vi "UMLEditor saveIniFileInfo.vi"(1 "localVariables":T2 {"ObjectHotspots"."HotSpot"."y" format="%.2f"; "ObjectHotspots"."HotSpot"."x" format="%.2f"; "NodesBounds"."height" format="%.2f"; "NodesBounds"."width" format="%.2f"; "NodesBounds"."y" format="%.2f"; "NodesBounds"."x" format="%.2f"; "offset"."y" format="%.2f"; "offset"."x" format="%.2f"; "gridSize" format="%.2f"; "dragStartBounds"."height" format="%.2f"; "dragStartBounds"."width" format="%.2f"; "dragStartBounds"."y" format="%.2f"; "dragStartBounds"."x" format="%.2f"; "dragStartPoint"."y" format="%.2f"; "dragStartPoint"."x" format="%.2f"; "rubberBandStart"."y" format="%.2f"; "rubberBandStart"."x" format="%.2f"; "lastMousePoint"."y" format="%.2f"; "lastMousePoint"."x" format="%.2f"; "zoom" format="%.2f"}, 5 "error in (no error)":errorcluster, 6 "diagramType":T1) -> (19 "error out":errorcluster)   [LabVIEW 2014]
doc: "Gets current diagram values"
uses:
  <resource>/Framework/Providers/Open_GDS/UML/UMLEditor/UMLEditor LocalVariablesType.ctl
  <resource>/Framework/Providers/Open_GDS/UML/Graphics_class/Graphics.lvclass
  <resource>/Framework/Providers/Open_GDS/UML/Grid_class/Grid.lvclass
  <resource>/Framework/Providers/Open_GDS/UML/AbstractEdge_class/AbstractEdge.lvclass
  <resource>/Framework/Providers/Open_GDS/UML/AbstractNode_class/AbstractNode.lvclass
  <resource>/Framework/Providers/Open_GDS/UML/UMLEditor/UMLEditor statesType.ctl
  <resource>/Framework/Providers/Open_GDS/UML/UMLEditor/UMLEditor tooltype.ctl
  <resource>/Framework/Providers/Open_GDS/UML/UMLEditor/UMLEditor toolsType.ctl
  <resource>/Framework/Providers/Open_GDS/UML/Graph_class/private/diagramType.ctl
  <resource>/Framework/Providers/Open_GDS/UML/Graph_class/Graph.lvclass
  <resource>/Framework/Providers/Open_GDS/UML/General/Point/Point Point2D.ctl
  <resource>/Framework/Providers/Open_GDS/UML/General/Rectangle/Rectangle Rectangle2D.ctl
  <resource>/Framework/Providers/Open_GDS/UML/UMLEditor/UMLEditor ExportType.ctl
  <resource>/Framework/Providers/Open_GDS/UML/UMLEditor/UMLEditor FlattenCommandType.ctl
  <resource>/Framework/Providers/Open_GDS/UML/UMLEditor/UMLEditor ExecuteCommandType.ctl
  <resource>/Framework/Providers/Open_GDS/UML/ContextHelp/ContextHelp_EventType.ctl
  <resource>/Framework/Providers/Open_GDS/UML/UMLEditor/UMLEditor_HotSpotData.ctl
  <resource>/Framework/Providers/Open_GDS/UML/UMLEditor/UMLEditor_HotSpotType.ctl
  <resource>/Framework/Providers/Open_GDS/UML/UmlEditor_class/EventData.ctl
  <resource>/Framework/Providers/Open_GDS/UML/UMLEditor/UMLEditor_IniFileData.ctl
  <resource>/Framework/Providers/Open_GDS/UML/UMLEditor/UMLEditor_SyncOptions.ctl
  <resource>/Framework/Providers/Open_GDS/UML/UMLEditor/UMLEditor_StoredPathes.ctl
  <resource>/Framework/Providers/Open_GDS/UML/UMLEditor/UMLEditor_StoredColors.ctl
  <resource>/Framework/Providers/Open_GDS/UML/UmlEditor_class/UmlEditor.lvclass
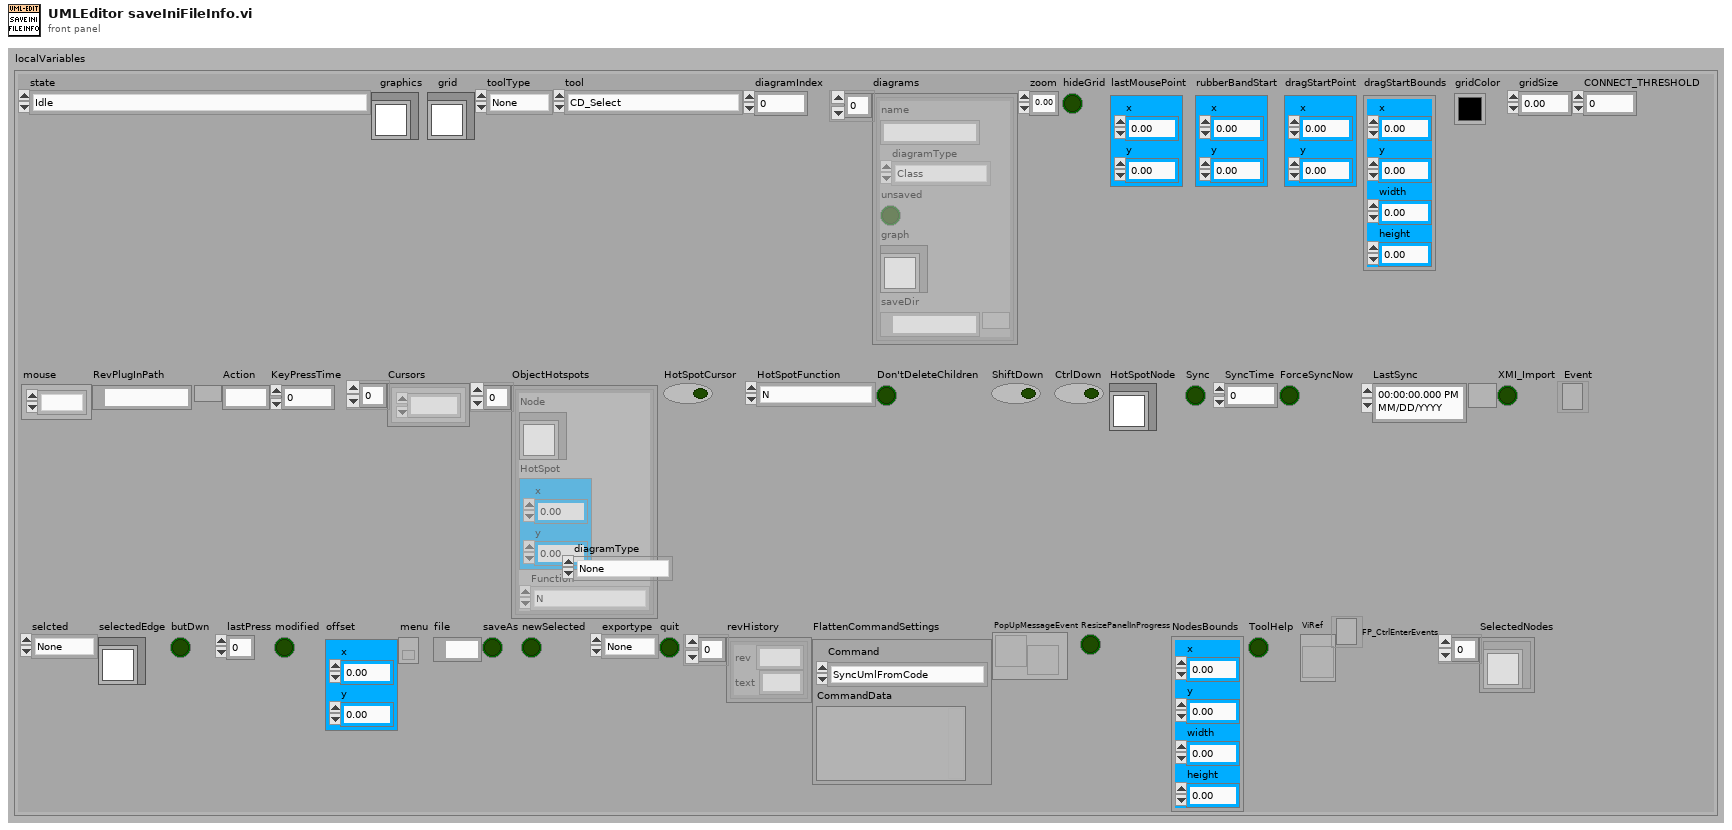
[diagram p1: front panel]
types:
  T1 = typedef "Graph.lvclass/diagramType.ctl" = enum16{"None", "Class", "Sequency", "State", "UseCase", "DQMH-Module"}
  T2 = typedef "UMLEditor LocalVariablesType.ctl" = cluster{"state":T3, "graphics":refnum<class "Graphics.lvclass">, "grid":refnum<class "Grid.lvclass">, "toolType":T4, "tool":T5, "diagramIndex":i32, "diagrams":cluster{"name":string, "diagramType":T1, "unsaved":bool, "graph":refnum<class "Graph.lvclass">, "saveDir":path}[], "zoom":dbl, "hideGrid":bool, "lastMousePoint":T6, "rubberBandStart":T6, "dragStartPoint":T6, "dragStartBounds":T7, "gridColor":u32, "gridSize":dbl, "CONNECT_THRESHOLD":i32, "selcted":T4, "selectedEdge":refnum<class "AbstractEdge.lvclass">, "butDwn":bool, "lastPress":u32, "modified":bool, "offset":T6, "menu":refnum<k9>, "file":path, "saveAs":bool, "newSelected":bool, "exportype":T8, "quit":bool, "revHistory":cluster{"rev":string, "text":string}[], "FlattenCommandSettings":T9, "PopUpMessageEvent":T11, "ResizePanelInProgress":bool, "NodesBounds":T7, "ToolHelp":bool, "ViRef":refnum<vi>, "FP_CtrlEnterEvents":refnum<event-registration>, "SelectedNodes":refnum<class "AbstractNode.lvclass">[], "mouse":refnum<k1>, "RevPlugInPath":path, "Action":string, "KeyPressTime":u32, "Cursors":refnum<k1>[], "ObjectHotspots":T12[], "HotSpotCursor":bool, "HotSpotFunction":T13, "Don'tDeleteChildren":bool, "ShiftDown":bool, "CtrlDown":bool, "HotSpotNode":refnum<class "AbstractNode.lvclass">, "Sync":bool, "SyncTime":u32, "ForceSyncNow":bool, "LastSync":timestamp, "XMI_Import":bool, "Event":refnum<event-registration>}
  T3 = typedef "UMLEditor statesType.ctl" = enum16{"Idle", "CheckLicense", "revHistory", "Init", "Init2", "EditSelected", "RemoveSelected", "PaintComponent", "ChangeZoom", "ChangeGridSize", "Open", "Close", "Save", "ExportPicture", "Export", "Repaint", "Error", "Exit", "QUIT", "CreateScript", "ExecuteScript", "ClassReversedEngineering", "PlugInReverseEngineering", "StateReversedEngineering", "AutoPlace", "ExecuteCommand", "OpenClass", "SyncAll", "StraightenAssociation", "Copy", "Paste", "AddNodeFromProjectTree", "AddNodeFromProjectTree+SyncAll", "PanAndRepaint", "Init3", "CopyPaste", "ApplyDesignPattern", "AnalyseViInStateDiagram", "AutoSync"}
  T4 = typedef "UMLEditor tooltype.ctl" = enum16{"None", "Node", "Edge"}
  T5 = typedef "UMLEditor toolsType.ctl" = enum16{"CD_Select", "CD_Class", "CD_Interface", "CD_Package", "CD_Note", "CD_Dependency", "CD_Inheritance", "CD_InterfaceImp", "CD_Association", "CD_Aggregation", "CD_Composite", "CD_NoteConn", "SQD_Select", "SQD_Object", "SQD_ActionBar", "SQD_Note", "SQD_Call", "SQD_NoteConn", "UD_Select", "UD_System", "UD_Actor", "UD_UseCase", "UD_Note", "UD_Assoiciation", "UD_Generalization", "UD_GeneralizationIncludes", "UD_GeneralizationExtends", "UD_Realization", "UD_Relationship", "UD_NoteEdge", "STD_Select", "STD_State", "STD_InitailState", "STD_FinalState", "STD_ChoiseState", "STD_StateTransation", "STD_Note", "STD_NoteEdge", "DM_Select", "DM_VI", "DM_Module", "DM_Request", "DM_RequestWait", "DM_Roundtrip", "DM_Broadcast", "DM_Note", "DM_NoteEdge"}
  T6 = typedef "Point Point2D.ctl" = cluster{"x":dbl, "y":dbl}
  T7 = typedef "Rectangle Rectangle2D.ctl" = cluster{"x":dbl, "y":dbl, "width":dbl, "height":dbl}
  T8 = typedef "UMLEditor ExportType.ctl" = enum16{"None", "Printer", "png", "jpg", "roseUML"}
  T9 = typedef "UMLEditor FlattenCommandType.ctl" = cluster{"Command":T10, "CommandData":variant}
  T10 = typedef "UMLEditor ExecuteCommandType.ctl" = enum16{"SyncUmlFromCode", "SyncCodeFromUML", "OpenClass", "OpenFile", "CreateClass", "CreateVI", "OpenClassAttribute", "LocateInProject"}
  T11 = typedef "ContextHelp_EventType.ctl" = refnum<user-event>
  T12 = typedef "UMLEditor_HotSpotData.ctl" = cluster{"Node":refnum<class "AbstractNode.lvclass">, "HotSpot":T6, "Function":T13}
  T13 = typedef "UMLEditor_HotSpotType.ctl" = enum16{"N", "NE", "E", "SE", "S", "SW", "W", "NW", "Expand", "Collaps"}
  T14 = typedef "UMLEditor_IniFileData.ctl" = cluster{"RecentFiles":string[], "LastDiagramType":T1, "ShowToolHelp":bool, "Paths":cluster{"LastSerachPath":path, "QueuedArrayStateVI":path, "ClassBasePath":path, "VITemplatePath":path, "ApplicationTemplatePath":path, "RevPlugIns":path}, "Colors":cluster{"ClassBackgroudColor":u32, "ClassBackgroudColorWithClassPath":u32, "ClassBackgroudColorForApplicationVIStereotype":u32, "ClassBackgroudColorForTypeStereotype":u32, "StateBackgroudColor":u32}, "ProjectBaseClassOption":bool, "CreateTypesWhenSynchronizing":bool, "AttributeToIgnoreInSync":string[], "ToolTip":cluster{"ToolTipOpen":bool, "LastToolTip":i32}, "ClassesToIgnoreInSync":string[], "UndoSize":i32, "OpenLastSavedFile":bool, "SyncOption":T15, "SyncTime":u32, "Params":cluster{"Name":string, "Value":string}[]}
  T15 = typedef "UMLEditor_SyncOptions.ctl" = cluster{"IgnoreInstrLib":bool, "IgnoreUserLib":bool, "IgnoreViLib":bool}
  T16 = typedef "UMLEditor_StoredPathes.ctl" = enum16{"LastSearchPath", "QueuedArrayStateVI", "ClassBasePath", "ViTemplatePath", "ApplicationTemplatePath", "IniFilePath", "WizDir", "RevPlugInPath"}
  T17 = typedef "UMLEditor_StoredColors.ctl" = enum16{"ClassBackgroudColor", "ClassBackgroudColorWithClassPath", "ClassBackgroudColorForApplicationVIStereotype", "ClassBackgroudColorForTypeStereotype", "StateBackgroudColor"}
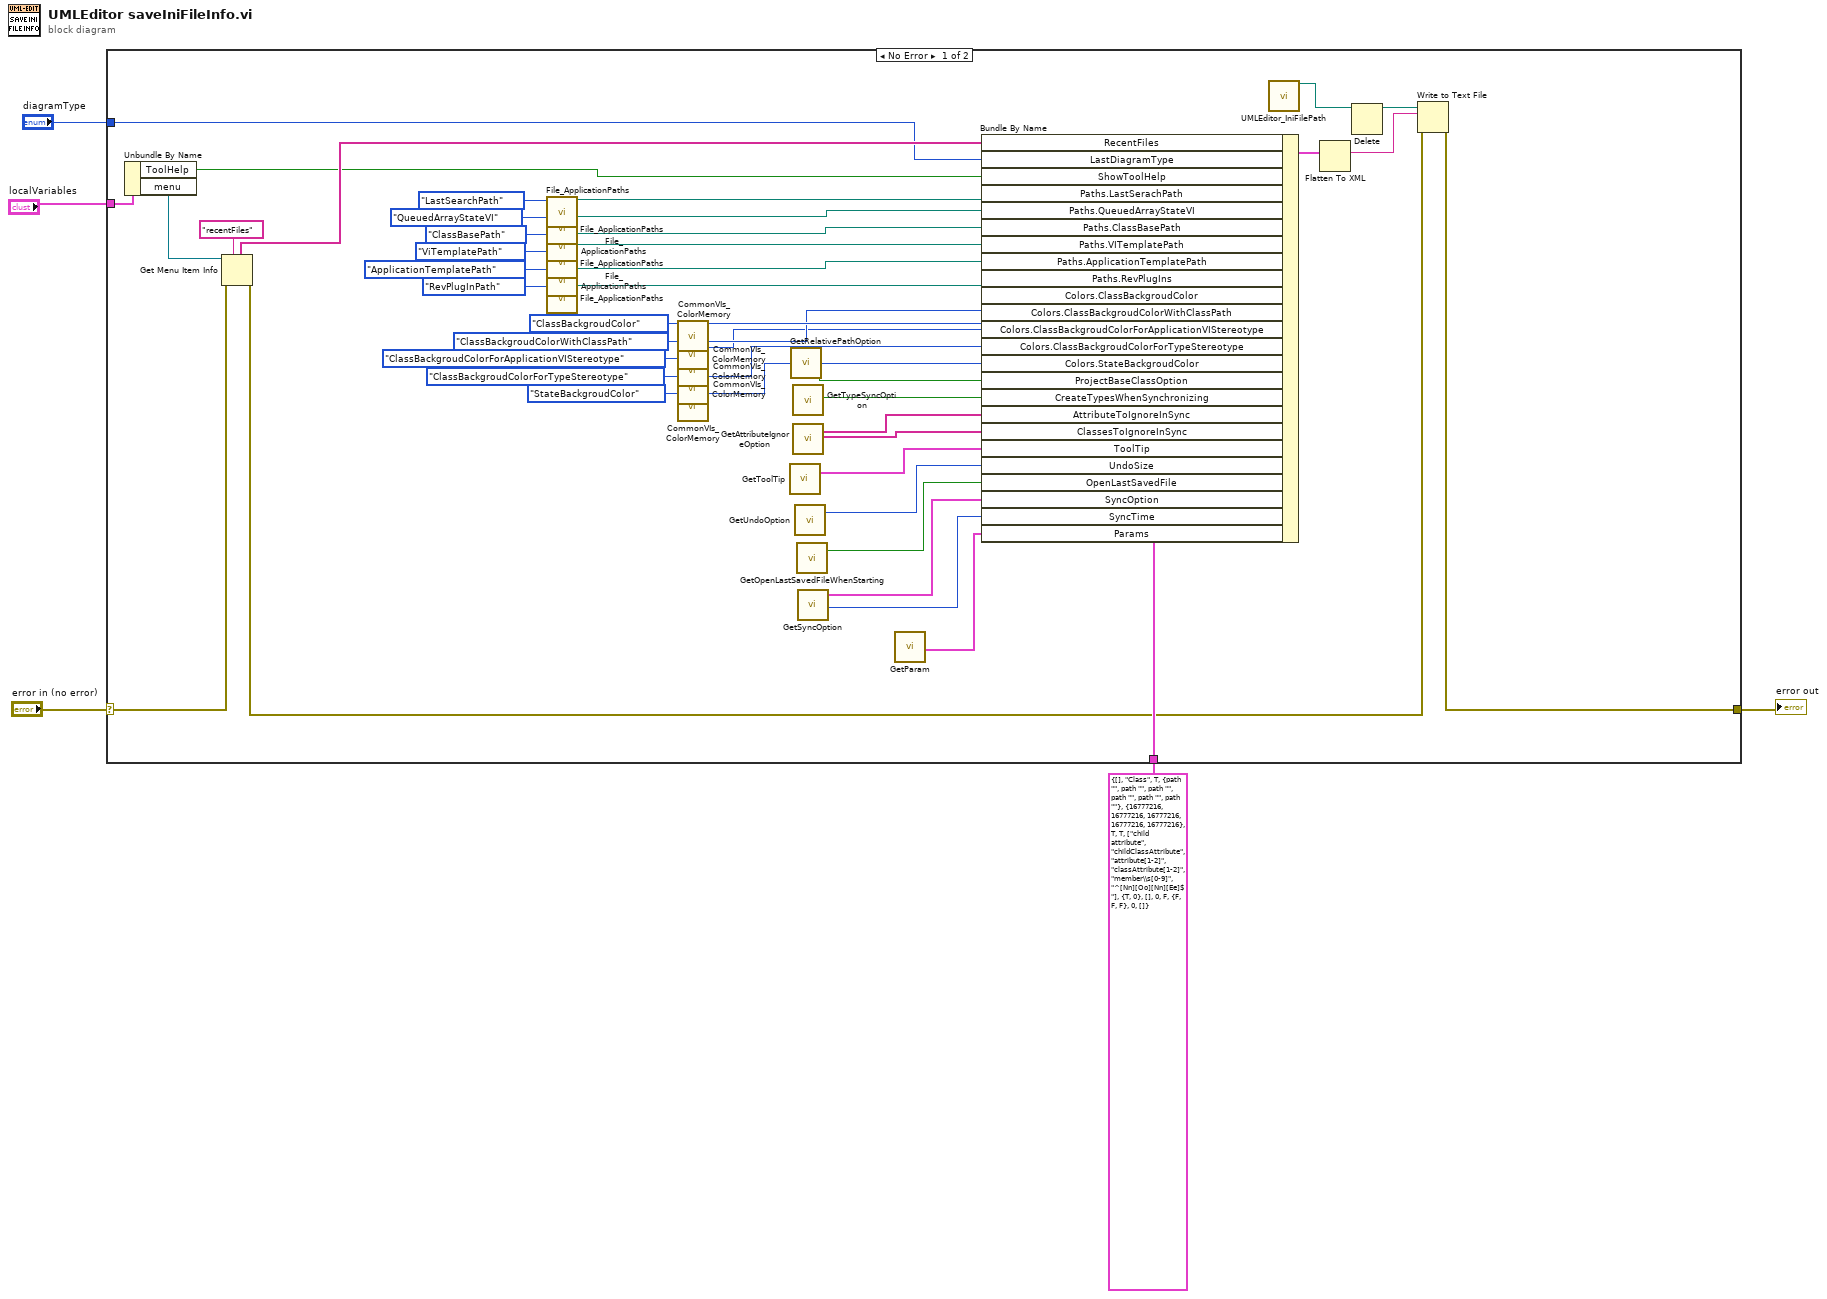
[diagram p0: block diagram]
diagram:
  n1 = case shown="No Error" "error in (no error)" {
    selector: "error in (no error)" -> [w48 w52]
    tunnel: [w14 w52] -> w4
    tunnel: "localVariables" -> [w51 _]
    tunnel: "diagramType" -> [w39 _]
    tunnel: T14 {"RecentFiles"=[], "LastDiagramType"=enum."Class", "ShowToolHelp"=TRUE, "Paths"={"LastSerachPath"=path "", "QueuedArrayStateVI"=path "", "ClassBasePath"=path "", "VITemplatePath"=path "", "ApplicationTemplatePath"=path "", "RevPlugIns"=path ""}, "Colors"={"ClassBackgroudColor"=16777216, "ClassBackgroudColorWithClassPath"=16777216, "ClassBackgroudColorForApplicationVIStereotype"=16777216, "ClassBackgroudColorForTypeStereotype"=16777216, "StateBackgroudColor"=16777216}, "ProjectBaseClassOption"=TRUE, "CreateTypesWhenSynchronizing"=TRUE, "AttributeToIgnoreInSync"=["child attribute", "childClassAttribute", "attribute[1-2]", "classAttribute[1-2]", "member\\s[0-9]", "^[Nn][Oo][Nn][Ee]$"], "ToolTip"={"ToolTipOpen"=TRUE, "LastToolTip"=0}, "ClassesToIgnoreInSync"=[], "UndoSize"=0, "OpenLastSavedFile"=FALSE, "SyncOption"={"IgnoreInstrLib"=FALSE, "IgnoreUserLib"=FALSE, "IgnoreViLib"=FALSE}, "SyncTime"=0, "Params"=[]} ("INiFileData") -> [w45 _]
    frame No Error {
      n2 = Unbundle By Name(w51) -> ("ToolHelp"=w38:bool, "menu"=w50:refnum<k9>)
      n3 = Get Menu Item Info(7:"recentFiles" ("item tag"), 8:w48, 11:w50) -> (0:w13:errorcluster, 5:w40:string[])  [unwired: 5 out]
      n4 = call <resource>:"File_ApplicationPaths.vi"("PathName"=UMLEditor_StoredPathes."LastSearchPath" ("UMLPathes")) -> ("Path Out"=w25:path)  [unwired: 3 in, 15 out]
      n5 = call <resource>:"File_ApplicationPaths.vi"("PathName"=UMLEditor_StoredPathes."QueuedArrayStateVI" ("UMLPathes")) -> ("Path Out"=w21:path)  [unwired: 3 in, 15 out]
      n6 = call <resource>:"File_ApplicationPaths.vi"("PathName"=UMLEditor_StoredPathes."ClassBasePath" ("UMLPathes")) -> ("Path Out"=w20:path)  [unwired: 3 in, 15 out]
      n7 = call <resource>:"File_ApplicationPaths.vi"("PathName"=UMLEditor_StoredPathes."ViTemplatePath" ("UMLPathes")) -> ("Path Out"=w19:path)  [unwired: 3 in, 15 out]
      n8 = call <resource>:"File_ApplicationPaths.vi"("PathName"=UMLEditor_StoredPathes."ApplicationTemplatePath" ("UMLPathes")) -> ("Path Out"=w17:path)  [unwired: 3 in, 15 out]
      n9 = call <resource>:"File_ApplicationPaths.vi"("PathName"=UMLEditor_StoredPathes."RevPlugInPath" ("UMLPathes")) -> ("Path Out"=w15:path)  [unwired: 3 in, 15 out]
      n10 = call <resource>:"CommonVIs_ColorMemory.vi"("ColorName"=UMLEditor_StoredColors."ClassBackgroudColor" ("UMLPathes")) -> ("Color Out"=w34:u32)  [unwired: 3 in, 15 out]
      n11 = call <resource>:"CommonVIs_ColorMemory.vi"("ColorName"=UMLEditor_StoredColors."ClassBackgroudColorWithClassPath" ("UMLPathes")) -> ("Color Out"=w29:u32)  [unwired: 3 in, 15 out]
      n12 = call <resource>:"CommonVIs_ColorMemory.vi"("ColorName"=UMLEditor_StoredColors."ClassBackgroudColorForApplicationVIStereotype" ("UMLPathes")) -> ("Color Out"=w28:u32)  [unwired: 3 in, 15 out]
      n13 = call <resource>:"CommonVIs_ColorMemory.vi"("ColorName"=UMLEditor_StoredColors."ClassBackgroudColorForTypeStereotype" ("UMLPathes")) -> ("Color Out"=w27:u32)  [unwired: 3 in, 15 out]
      n14 = call <resource>:"CommonVIs_ColorMemory.vi"("ColorName"=UMLEditor_StoredColors."StateBackgroudColor" ("UMLPathes")) -> ("Color Out"=w26:u32)  [unwired: 3 in, 15 out]
      n15 = call <resource>:"GetToolTip.vi"() -> ("ToolTip"=w12:cluster{"ToolTipOpen":bool, "LastToolTip":i32})  [unwired: 1 in, 18 out]
      n16 = call <resource>:"GetRelativePathOption.vi"() -> ("UseProjectFolderAsBasePath"=w36:bool)  [unwired: 1 in, 18 out]
      n17 = call <resource>:"GetTypeSyncOption.vi"() -> ("TypeSyncOption"=w35:bool)  [unwired: 1 in, 18 out]
      n18 = call <resource>:"GetAttributeIgnoreOption.vi"() -> ("Attr"=w37:string[], "ClassesToIgnore"=w11:string[])  [unwired: 1 in, 17 out]
      n19 = call <resource>:"GetUndoOption.vi"() -> ("UndoSize"=w10:i32)  [unwired: 1 in, 18 out]
      n20 = call <resource>:"GetOpenLastSavedFileWhenStarting.vi"() -> ("OpenLastSavedFileWhenStarting"=w9:bool)  [unwired: 18 in, 1 out]
      n21 = call <resource>:"GetSyncOption.vi"() -> ("SyncOption"=w8:T15, "SyncTime(s)"=w7:i32)  [unwired: 17 in, 1 out]
      n22 = call <resource>:"GetParam.vi"() -> ("Array"=w6:cluster{string, "Value":string}[])  [unwired: 17 in, 2 out]
      n23 = Bundle By Name(cluster=w45, "RecentFiles"=w40, "LastDiagramType"=w39, "ShowToolHelp"=w38, "Paths.LastSerachPath"=w25, "Paths.QueuedArrayStateVI"=w21, "Paths.ClassBasePath"=w20, "Paths.VITemplatePath"=w19, "Paths.ApplicationTemplatePath"=w17, "Paths.RevPlugIns"=w15, "Colors.ClassBackgroudColor"=w34, "Colors.ClassBackgroudColorWithClassPath"=w29, "Colors.ClassBackgroudColorForApplicationVIStereotype"=w28, "Colors.ClassBackgroudColorForTypeStereotype"=w27, "Colors.StateBackgroudColor"=w26, "ProjectBaseClassOption"=w36, "CreateTypesWhenSynchronizing"=w35, "AttributeToIgnoreInSync"=w37, "ClassesToIgnoreInSync"=w11, "ToolTip"=w12, "UndoSize"=w10, "OpenLastSavedFile"=w9, "SyncOption"=w8, "SyncTime"=w7, "Params"=w6) -> (w42:T14)
      n24 = call <resource>:"UMLEditor_IniFilePath.vi"() -> ("Get Path"=w41:path)  [unwired: 2 in, 17 out]
      n25 = Flatten To XML(anything=w42) -> (xml string=w44:string)
      n26 = Delete(path (use dialog)=w41) -> (deleted path=w43:path)  [unwired: 1 in, 5 out]
      n27 = Write to Text File(file (use dialog)=w43, text=w44, error in=w13) -> (error out=w14:errorcluster)  [unwired: 3 out]
    }
    frame Error {
    }
  }
  "error out" <- w4
